vi "Test shm get Event scalars LV.vi"(8 "error in (no error)":errorcluster, 11 "logevent_scalars_Ctl":T1) -> (0 "error out":errorcluster, 2 "function return":i32, 3 "logevent_scalars_Ctl out":T1)   [LabVIEW 2018, in "SALLV_Test.lvlib"]
doc: "int Test_shm_getEvent_scalarsLV(Test_logevent_scalarsLV *logevent_scalars_Ctl );"
uses:
  SALLV_Test.lvlib
  SALLV_Test.so
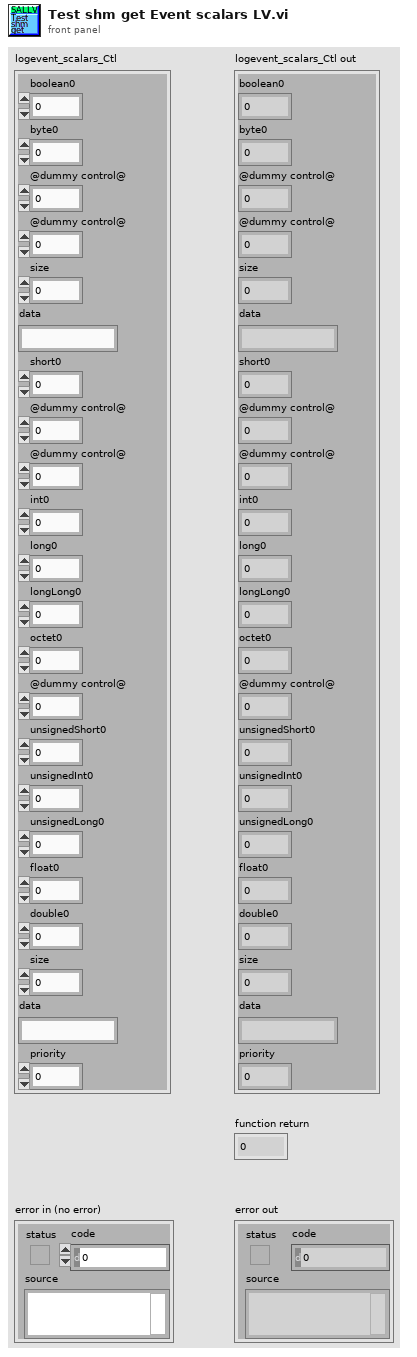
[diagram p1: front panel]
types:
  T1 = cluster{"boolean0":u8, "byte0":u8, "@dummy control@":i8, "@dummy control@":i8, "size":i32, "data":string, "short0":i16, "@dummy control@":i8, "@dummy control@":i8, "int0":i32, "long0":i32, "longLong0":i32, "octet0":u8, "@dummy control@":i8, "unsignedShort0":u16, "unsignedInt0":u32, "unsignedLong0":u32, "float0":sgl, "double0":dbl, "size":i32, "data":string, "priority":i32}
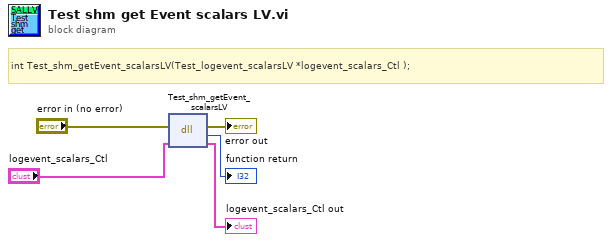
[diagram p0: block diagram]
diagram:
  # "int Test_shm_getEvent_scalarsLV(Test_logevent_scalarsLV *logevent_scalars_Ctl );"
  n1 = dll-call lib="home/ttsai/Documents/salLabVIEWtestData/SALLV_Test.*" fn="Test_shm_getEvent_scalarsLV"(error in="error in (no error)", "logevent_scalars_Ctl"="logevent_scalars_Ctl") -> (error out=→"error out":errorcluster, →"function return":i32, "logevent_scalars_Ctl"=→"logevent_scalars_Ctl out":T1)  [unwired: 2 in, 1 out]
